vi "FPGA_controlled VI.vi"() -> ()   [LabVIEW 2020]
uses:
  <vilib>/rvi/Emulation/niFpgaGetClockAttributes.vi
  <vilib>/rvi/Emulation/niFpgaSctlEmulationGetInTimedLoop.vi
  <vilib>/rvi/Emulation/niFpgaEmulationReportErrorSimple.vi
  <vilib>/rvi/eio/common/nirviEmuTemplateMethod_errors.vi
  <vilib>/rvi/Emulation/niFpgaCriticalErrorInLSC.vi
  <vilib>/eio/EIONode/EIONode.xnode
panel:
  out "Mod1/AI0":fxp<+/-,26,5>
  in  "stop":bool
  in  "Mod4/AO0":fxp<+/-,20,5>
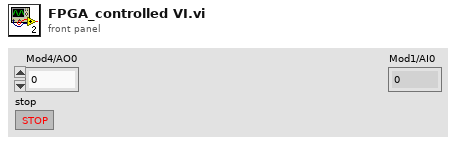
[diagram p1: front panel]
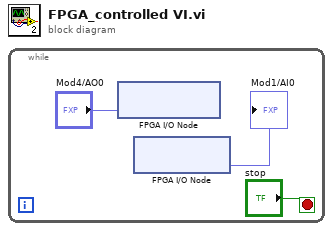
[diagram p0: block diagram]
diagram:
  n1 = while {
    stop <- "stop" stop-if-true
    n2 = xnode "FPGA I/O Node"("Mod4/AO0"="Mod4/AO0") -> ()  [unwired: 1 in, 1 out]
    n3 = xnode "FPGA I/O Node"() -> ("Mod1/AI0"=→"Mod1/AI0":fxp<+/-,26,5>)  [unwired: 1 in, 1 out]
  }
